vi "Read Response.vi"(8 "error in":errorcluster, 11 "Kronos in":refnum<class "Kronos.lvclass">) -> (0 "error out":errorcluster, 3 "Kronos out":refnum<class "Kronos.lvclass">)   [LabVIEW 2017, in "Kronos.lvlib" / "Kronos.lvclass"]
uses:
  Kronos.lvclass
  builds/Built/Laser.lvlibp/Laser.lvclass
  C:/Users/Ron.Dexter.LUMINARTECH/Desktop/builds/Built/Laser.lvlibp/Laser.lvclass
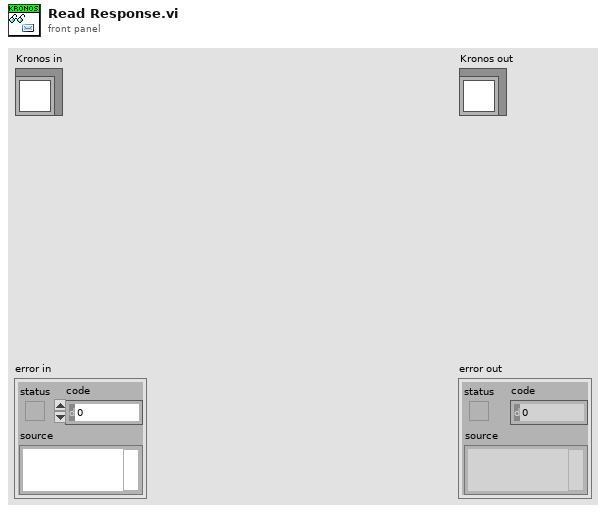
[diagram p1: front panel]
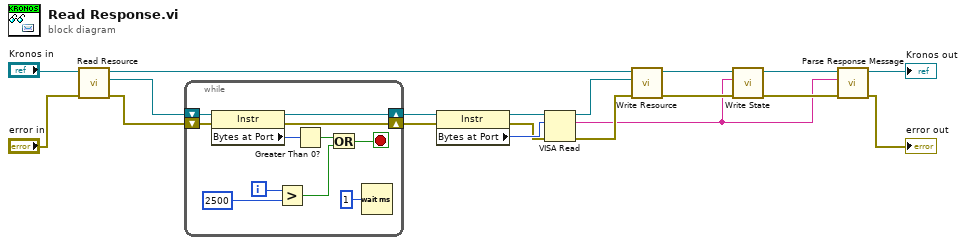
[diagram p0: block diagram]
diagram:
  n1 = call "Read Resource.vi"("error in (no error)"="error in", "Laser in"="Kronos in") -> ("error out"=w16:errorcluster, "Resource"=w17:refnum<visa-resource-name>, "Laser out"=w8:refnum<class "Kronos.lvclass">)  [unwired: 7 in]
  n2 = while {
    shift-right: [w23] -> w12
    shift-left: w17 -> [w30]
    shift-right: [w22] -> w6
    shift-left: w16 -> [w21]
    i -> [w27]
    stop <- w24 stop-if-true
    n3 = property class="Instr"(reference=w30, error in=w21) -> (reference out=w23:refnum<visa-resource-name>, error out=w22:errorcluster, "Bytes at Port"=w29:u32)
    n4 = Greater?(x=w27, y=2500) -> (0:w25:bool)
    n5 = Greater Than 0?(x=w29) -> (x > 0?=w28:bool)
    n6 = Or(x=w28, y=w25) -> (x .or. y?=w24:bool)
    n7 = Wait (ms)(milliseconds to wait=u32 1) -> ()  [unwired: 1 out]
  }
  n8 = property class="Instr"(reference=w12, error in=w6) -> (reference out=w13:refnum<visa-resource-name>, error out=w14:errorcluster, "Bytes at Port"=w15:u32)
  n9 = VISA Read(VISA resource name=w13, byte count=w15, error in (no error)=w14) -> (VISA resource name out=w11:refnum<visa-resource-name>, read buffer=w1:string, error out=w10:errorcluster)  [unwired: 1 out]
  n10 = call "Write Resource.vi"("error in (no error)"=w10, "Resource"=w11, "Laser in"=w8) -> ("error out"=w4:errorcluster, "Laser out"=w5:refnum<class "Kronos.lvclass">)  [unwired: 7 in]
  n11 = call "Write State.vi"("error in (no error)"=w4, "State"=w1, "Laser in"=w5) -> ("error out"=w3:errorcluster, "Laser out"=w2:refnum<class "Kronos.lvclass">)  [unwired: 7 in]
  n12 = call "Parse Response Message.vi"("error in"=w3, "Response"=w1, "Kronos in"=w2) -> ("error out"=→"error out":errorcluster, "Kronos out"=→"Kronos out":refnum<class "Kronos.lvclass">)  [unwired: 7 in]
